vi "configuration UI.vi"() -> ()   [LabVIEW 2014, in "OPC UA Client editor node.lvclass"]
uses:
  OPC UA Client editor node.lvclass
  <vilib>/NI/Configuration Framework/Node/NodeRef.ctl
  <vilib>/NI/Configuration Framework/Node/NISE_CEF_Node.lvclass
  <vilib>/NI/AMC/Message Queue.ctl
  <vilib>/NI/AMC/Message.ctl
  <vilib>/NI/Tools/Keyed Array/KeyedArray.ctl
  <vilib>/NI/Configuration Framework/Node/UserEventRef.ctl
  <vilib>/NI/Configuration Framework/Controls/EventCluster.ctl
  <vilib>/NI/DCAF UI Toolkit/Controls/Configure.ctl
  <vilib>/NI/DCAF UI Toolkit/Controls/Add.ctl
  <vilib>/NI/DCAF UI Toolkit/Controls/Remove.ctl
  <vilib>/NI/Configuration Framework/Node/StopEvent.ctl
  <vilib>/NI/Configuration Framework/Node/RefreshUIEvent.ctl
  <vilib>/NI/Configuration Framework/Node/CacheState.ctl
  <vilib>/NI/Configuration Framework/Node/NodeChangeEvent.ctl
  <vilib>/NI/Tag Bus/tag/Data Type.ctl
  Permissions Enum.ctl
  <vilib>/NI/DCAF/Tag Editor Core/Table API/Available Tag Menu/channel action event.ctl
  <vilib>/NI/DCAF/Tag Editor Core/Table API/Available Tag Menu/dialog output action.ctl
  <vilib>/NI/Tag Bus Module Framework/channel/TBM channel.lvclass
  <vilib>/NI/Tag Bus/tag/tag descriptor.lvclass
  <vilib>/NI/DCAF/Tag Editor Core/Table API/Table Manager/Call Back Ref Type Def.ctl
  <vilib>/NI/DCAF/Tag Editor Core/Configuration Editor/Classes/Engine Parent/Engine Parent Editor Node.lvclass
  <vilib>/NI/DCAF/Tag Editor Core/Configuration Editor/Classes/Module editor node/module editor node.lvclass
  OPC UA DataType Enum.ctl
  <vilib>/NI/DCAF/Tag Editor Core/Table API/Table Manager/references.ctl
  module/configuration/OPC UA Client configuration.lvclass
  module/configuration/OPC UA Client configuration.lvclass/OPC UA Client configuration.ctl
  OPC UA Client editor node.lvclass/OPC UA Client editor node.ctl
  module/configuration/Read Connection Configuration.vi
  module/configuration/Write Connection Configuration.vi
  <vilib>/NI/Configuration Framework/serializable configuration/NISE_CEF_serializable configuration.lvclass
  <vilib>/NI/DCAF/Tag Editor Core/Table API/Listbox/Multi Column Listbox.lvclass
  <vilib>/NI/Configuration Framework/NISE_CEF_TreeControl.lvlib
  <vilib>/NI/Tools/Keyed Array/Tools_KeyedArray.lvlib
  <vilib>/NI/AMC/AMC.lvlib
  <vilib>/NI/DCAF/Tag Editor Core/Table API/Table Manager.lvlib
  <vilib>/NI/DCAF/Tag Editor Core/Table API/Table Manager/Table Manager.lvclass
  <vilib>/NI/DCAF UI Toolkit/Controls/DCAF UI Elements.lvlib
panel:
  in  "OPC Data Type":T1
  in  "user event out":refnum<user-event>
  in  "Permissions":T2
  in  "data type":T3
  in  "node change":T4
  in  "cache state":T5
  in  "refresh UI":T6
  in  "stop event":T7
  in  "Tab Control":enum32{"Nodes", "Client Configuration"}(tab)
  in  "Remove Button":T8
  in  "Add Button":T9
  in  "Table":i32(listbox)
  in  "settings":T10
  in  "ClientCert.Relative?":bool
  in  "ServerCerts.Relative?":bool
  in  "Server Certificate Paths":string[](array[string])
  in  "Client Certificate Path":string
  in  "Server Endpoint URL":string
  in  "Username/Password":cluster{"Username":string, "Password":string}
  in  "Security Policy":T11
  in  "user event":T12
  in  "main queue":T13
  in  "node ref":T14
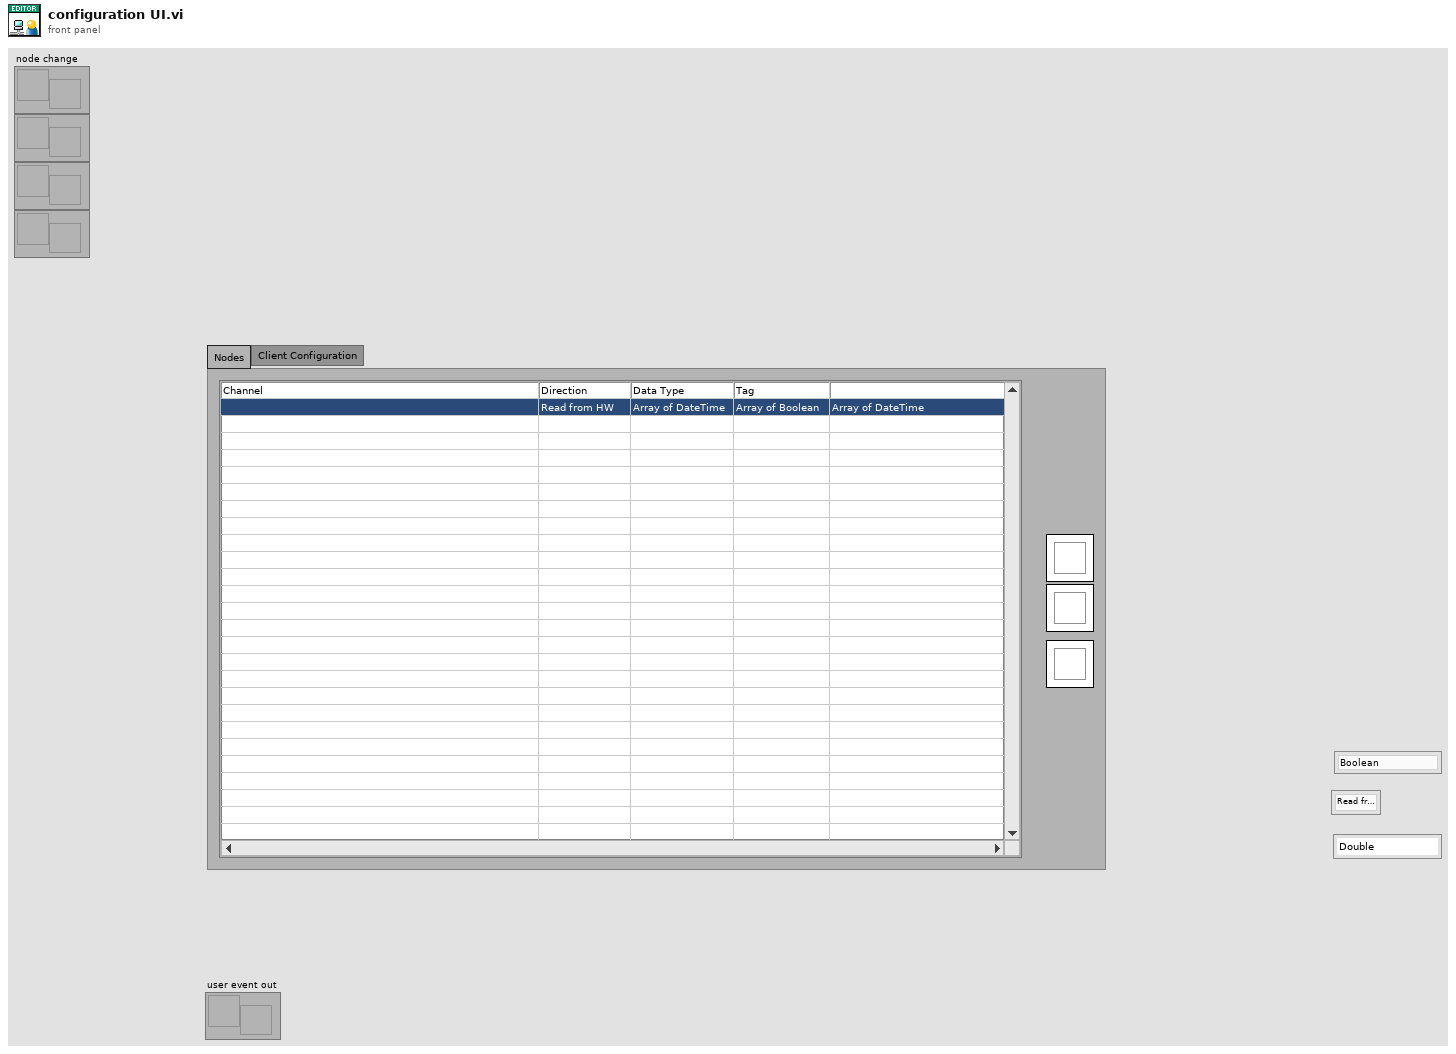
[diagram p1: front panel]
types:
  T1 = typedef "OPC UA Client editor node.lvclass/OPC UA DataType Enum.ctl" = enum16{"Boolean", "SByte", "Byte", "Int16", "UInt16", "Int32", "UInt32", "Int64", "UInt64", "Float", "Double", "String", "DateTime", "ByteString", "Array of Boolean", "Array of SByte", "Array of Byte", "Array of Int16", "Array of UInt16", "Array of Int32", "Array of UInt32", "Array of Int64", "Array of UInt64", "Array of Float", "Array of Double", "Array of String", "Array of DateTime"}
  T2 = typedef "OPC UA Client editor node.lvclass/Permissions Enum.ctl" = enum16{"Read from HW", "Write to HW"}
  T3 = typedef "tag bus.lvlib/tag descriptor.lvclass/Data Type.ctl" = enum16{"Double", "Single", "I64", "I32", "I16", "I8", "U64", "U32", "U16", "U8", "Boolean", "String", "Array of Double", "Array of Single", "Array of I64", "Array of I32", "Array of I16", "Array of I8", "Array of U64", "Array of U32", "Array of U16", "Array of U8", "Array of Boolean", "Array of String"}
  T4 = typedef "NISE_CEF_Node.lvclass/NodeChangeEvent.ctl" = refnum<user-event>
  T5 = typedef "NISE_CEF_Node.lvclass/CacheState.ctl" = refnum<user-event>
  T6 = typedef "NISE_CEF_Node.lvclass/RefreshUIEvent.ctl" = refnum<user-event>
  T7 = typedef "NISE_CEF_Node.lvclass/StopEvent.ctl" = refnum<user-event>
  T8 = typedef "DCAF UI Elements.lvlib/Remove.ctl" = bool
  T9 = typedef "DCAF UI Elements.lvlib/Add.ctl" = bool
  T10 = typedef "DCAF UI Elements.lvlib/Configure.ctl" = bool
  T11 = cluster{"Message Mode":enum16{"None", "Sign", "Sign and Encrypt"}, "Security":enum16{"Basic256", "Basic128Rsa15"}}
  T12 = typedef "NISE_CEF_Node.lvclass/UserEventRef.ctl" = refnum<user-event>
  T13 = typedef "AMC.lvlib/Message Queue.ctl" = refnum<queue>
  T14 = typedef "NISE_CEF_Node.lvclass/NodeRef.ctl" = refnum<data-value>
  T15 = typedef "Table Manager.lvlib/Table Manager.lvclass/references.ctl" = cluster{"stop event":T7, "refresh UI":T6, "cache state":T5, "node change":T4, "user event out":refnum<user-event>, "main queue":T13, "user event":T12}
  T16 = typedef "Table Manager.lvlib/Table Manager.lvclass/object ref.ctl" = cluster{"engine":refnum<data-value>, "Node Ref":refnum<data-value>}
  T17 = typedef "OPC UA Client configuration.lvclass/Client Connection Configuration.ctl" = cluster{"Server Certificates":cluster{"Relative Path?":bool, "Server Paths":string[]}, "Client Certificates":cluster{"Relative Path?":bool, "Client Path":string}, "Client Configuration":cluster{"Server Endpoint URL":string, "Security Policy":cluster{"Message Mode":enum16{"None", "Sign", "Sign and Encrypt"}, "Security":enum16{"Basic256", "Basic128Rsa15"}}, "Username/Password":cluster{"Username":string, "Password":string}}}
  T18 = typedef "Table Manager.lvlib/Column.lvclass/Column Descriptor.ctl" = cluster{"name":string, "caption":string, "Column Type":T19, "Params":string, "AutoSizeMode":i32, "FillWeight":sgl, "MinWidth":u32, "tooltip":string, "Enum Reference":refnum<vi>, "Channel suffix":string, "Read Only":bool, "Call Back VI":T20, "DT Dependency":i32, "name dependency":i32, "data type":T3, "Custom Column":refnum<class "Column.lvclass">}
  T19 = typedef "Table Manager.lvlib/Column.lvclass/Column Type.ctl" = enum16{"String", "Mapping", "Enum", "Custom"}
  T20 = typedef "Table Manager.lvlib/Table Manager.lvclass/Call Back Ref Type Def.ctl" = refnum<vi>
  T21 = typedef "Table Manager.lvlib/Table Manager.lvclass/Table Events.ctl" = cluster{"Menu Selection":refnum<user-event>}
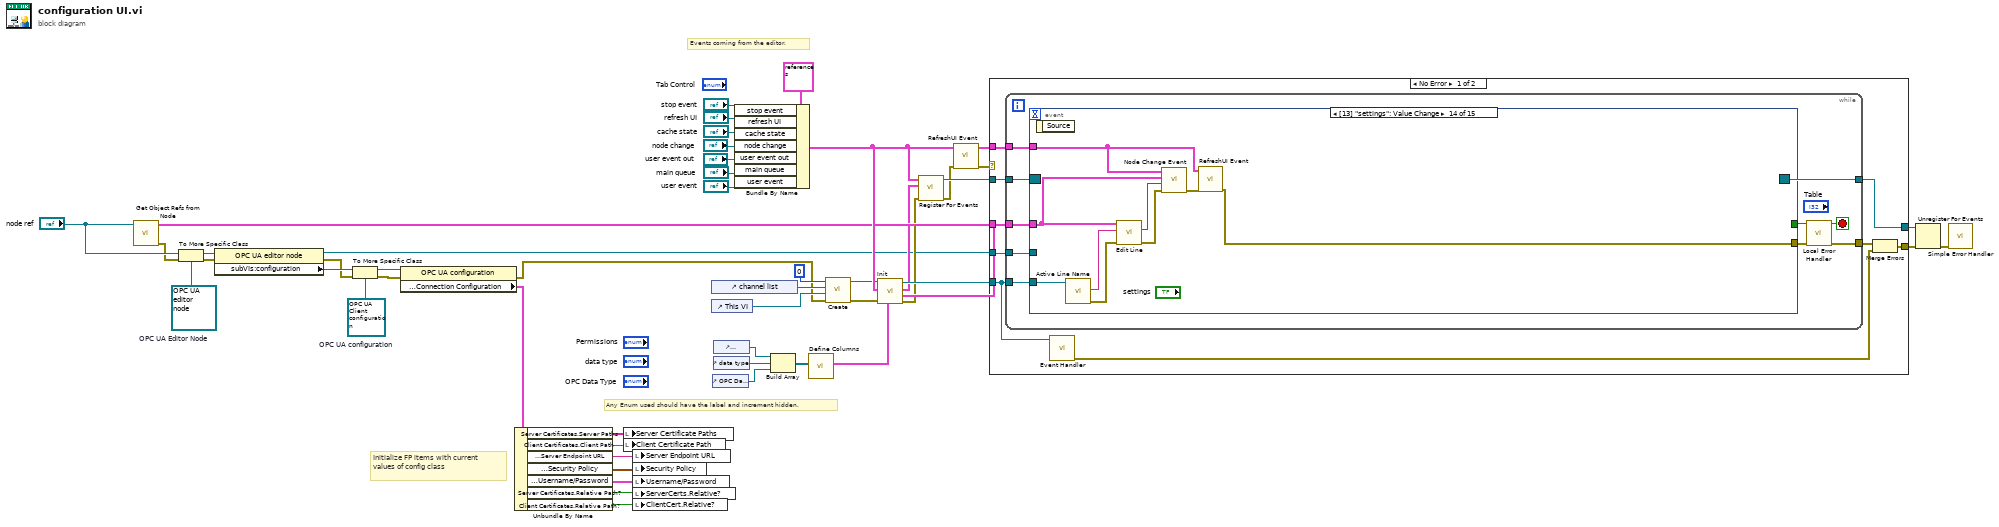
[diagram p0: block diagram]
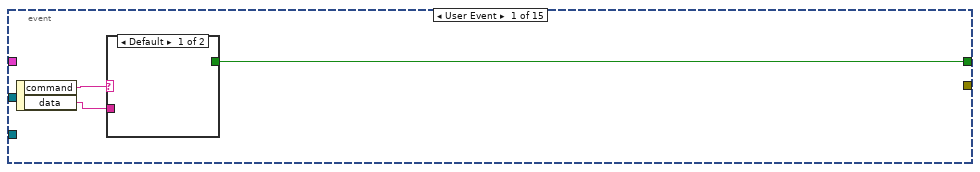
[diagram p2: hidden frame]
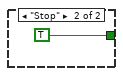
[diagram p3: hidden frame]
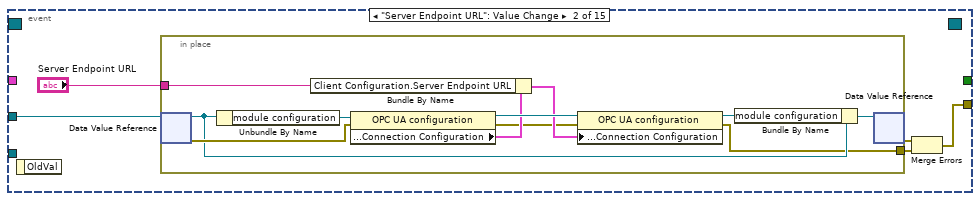
[diagram p4: hidden frame]
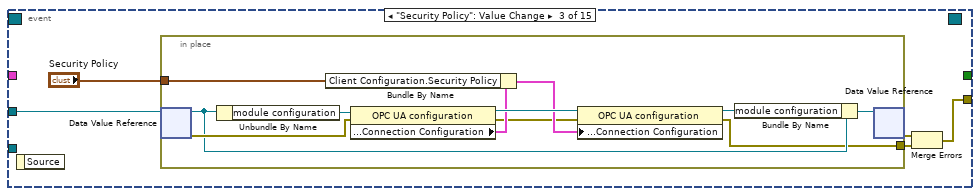
[diagram p5: hidden frame]
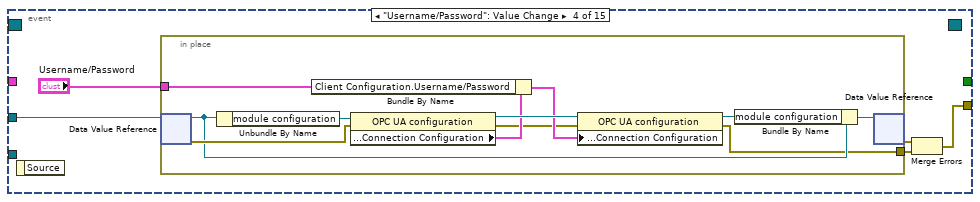
[diagram p6: hidden frame]
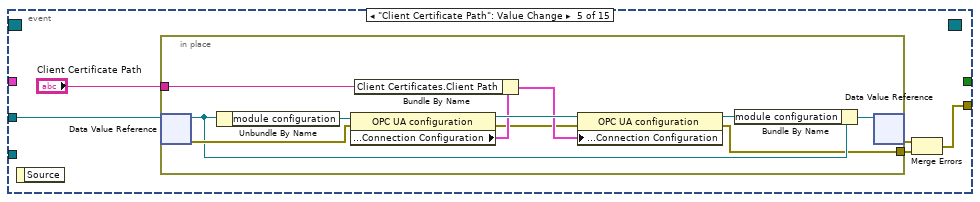
[diagram p7: hidden frame]
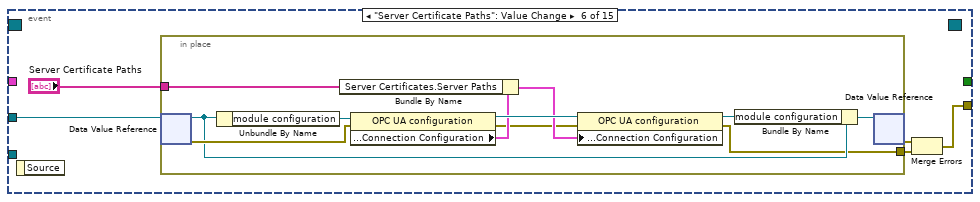
[diagram p8: hidden frame]
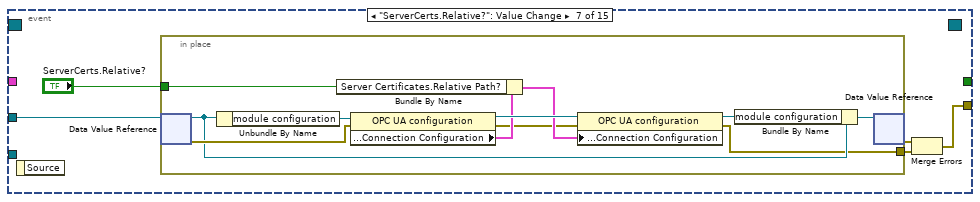
[diagram p9: hidden frame]
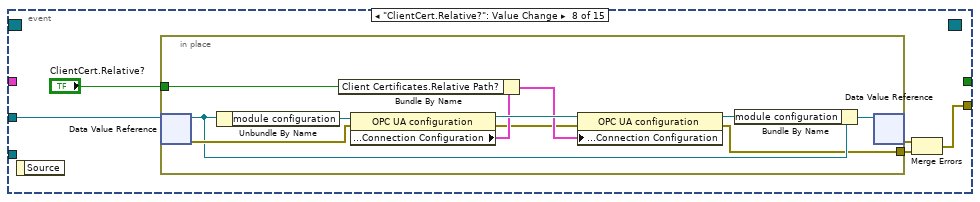
[diagram p10: hidden frame]
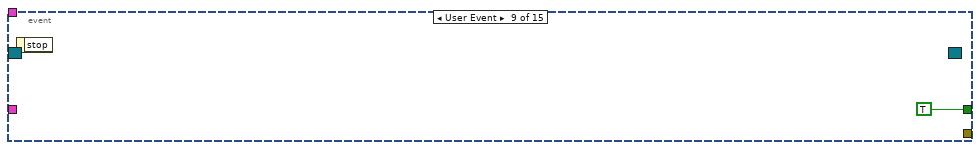
[diagram p11: hidden frame]
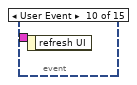
[diagram p12: hidden frame]
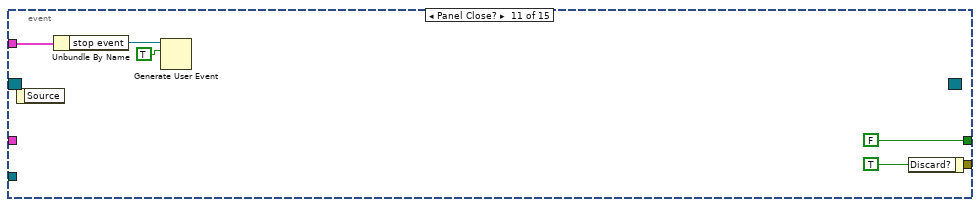
[diagram p13: hidden frame]
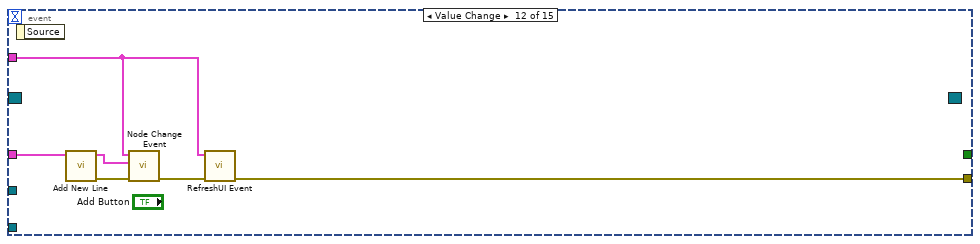
[diagram p14: hidden frame]
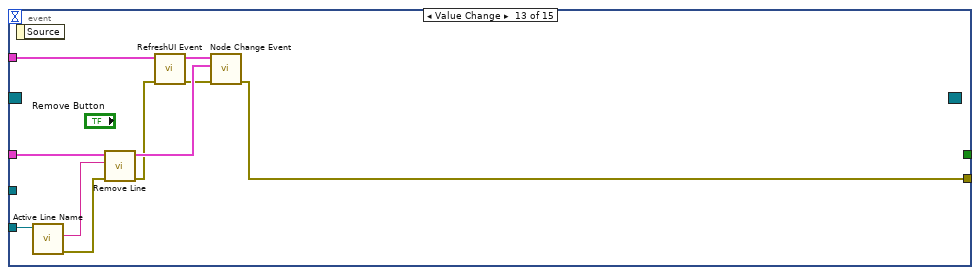
[diagram p15: hidden frame]
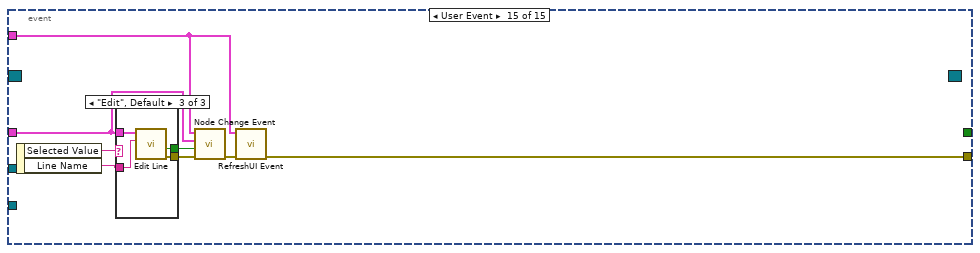
[diagram p16: hidden frame]
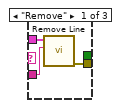
[diagram p17: hidden frame]
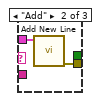
[diagram p18: hidden frame]
diagram:
  w11 = refnum<class "OPC UA Client configuration.lvclass"> refnum  # OPC UA configuration
  w19 = refnum<data-value> refnum  # OPC UA Editor Node
  # "Initialize FP items with current values of config class"
  # "Any Enum used should have the label and increment hidden."
  # "Events coming from the editor."
  n1 = call "Get Object Refs from Node.vi"("Data Value Reference in"="node ref") -> ("error out"=w18:errorcluster, "references"=w32:T16)  [unwired: 9 in]
  n2 = To More Specific Class(target class=w19, reference="node ref", error in=w18) -> (specific class reference=w16:refnum<data-value>, error out=w17:errorcluster)
  n3 = property class="OPC UA editor node"(reference=w16, error in=w17) -> (reference out=w15:refnum<data-value>, error out=w9:errorcluster, "subVIs:configuration"=w14:refnum<class "NISE_CEF_serializable configuration.lvclass">)
  n4 = To More Specific Class(target class=w11, reference=w14, error in=w9) -> (specific class reference=w13:refnum<class "OPC UA Client configuration.lvclass">, error out=w12:errorcluster)
  n5 = property class="OPC UA configuration"(reference=w13, error in=w12) -> (error out=w8:errorcluster, "Customize:Properties:Connection Configuration"=w10:T17)  [unwired: 1 out]
  n6 = Unbundle By Name(w10) -> ("Server Certificates.Server Paths"=w6:string[], "Client Certificates.Client Path"=w5:string, "Client Configuration.Server Endpoint URL"=w2:string, "Client Configuration.Security Policy"=w3:T11, "Client Configuration.Username/Password"=w4:cluster{"Username":string, "Password":string}, "Server Certificates.Relative Path?"=w50:bool, "Client Certificates.Relative Path?"=w1:bool)
  n7 = local write "Server Certificate Paths"(w6) -> ()
  n8 = local write "Client Certificate Path"(w5) -> ()
  n9 = local write "Server Endpoint URL"(w2) -> ()
  n10 = local write "Security Policy"(w3) -> ()
  n11 = local write "Username/Password"(w4) -> ()
  n12 = local write "ServerCerts.Relative?"(w50) -> ()
  n13 = local write "ClientCert.Relative?"(w1) -> ()
  n14 = control-ref of="channel list"() -> (w25:refnum<vi>)
  n15 = control-ref of="This VI"() -> (w23:refnum<vi>)
  n16 = control-ref of="OPC Data Type"() -> (w21:refnum<vi>)
  n17 = control-ref of="Permissions"() -> (w35:refnum<vi>)
  n18 = control-ref of="data type"() -> (w34:refnum<vi>)
  n19 = Bundle By Name(cluster=T15 {"stop event"=refnum, "refresh UI"=refnum, "cache state"=refnum, "node change"=refnum, "user event out"=refnum, "main queue"=refnum, "user event"=refnum} ("References"), "stop event"="stop event", "refresh UI"="refresh UI", "cache state"="cache state", "node change"="node change", "user event out"="user event out", "main queue"="main queue", "user event"="user event") -> (w36:T15)
  n20 = Build Array(w35, w34, w21) -> (w33:refnum<vi>[])
  n21 = call "Define Columns.vi"("Enum Array"=w33) -> ("Column Definition"=w38:T18[])  [unwired: 10 in]
  n22 = call <vilib>:"Create.vi"("error in (no error)"=w8, "Top VI"=w23, "Listbox"=w25, "Index"=0) -> ("error out"=w7:errorcluster, "reference out"=w22:refnum<class "Multi Column Listbox.lvclass">)  [unwired: 6 in]
  n23 = call-dynamic "Init.vi"("Column Descriptors"=w38, "error in (no error)"=w7, "Node object refs"=w32, "Event References"=w36, "Multi Column Listbox in"=w22) -> ("error out"=w27:errorcluster, "Table Events"=w26:T21, "Multi Column Listbox out"=w31:refnum<class "Multi Column Listbox.lvclass">)  [unwired: 4 in]
  n24 = call "Register For Events.vi"("error in"=w27, "Table Events"=w26, "References"=w36) -> ("error out"=w29:errorcluster, "Event Registration Refnum"=w39:refnum<event-registration>)  [unwired: 7 in]
  n25 = call "RefreshUI Event.vi"("error in (no error)"=w29, "References in"=w36) -> ("error out"=w28:errorcluster, "References out"=w37:T15)  [unwired: 8 in]
  n26 = case shown="No Error" w28 {
    selector: w28 -> [_ w233]
    tunnel: w39 -> [w59 w232]
    tunnel: [w58 w232] -> w49
    tunnel: [w52 w233] -> w48
    tunnel: w37 -> [w57 _]
    tunnel: w32 -> [w56 _]
    tunnel: w31 -> [w55 _]
    tunnel: w15 -> [w51 _]
    frame No Error {
      n27 = while {
        tunnel: w59 -> [w69]
        tunnel: [w68] -> w58
        tunnel: [w65] -> w53
        tunnel: w57 -> [w63]
        tunnel: w56 -> [w62]
        tunnel: w55 -> [w61]
        tunnel: w51 -> [w60]
        stop <- w67 stop-if-true
        n28 = event shown="[13] \"settings\": Value Change" {
          selector: w69 -> [_ _ _ _ _ _ _ _ _ _ _ _ _ _ _]
          dyn-events: [_ _ _ _ _ _ _ _ _ _ _ _ _ _ _] -> w68
          timeout: _ -> [_ _ _ _ _ _ _ _ _ _ _ _ _ _ _]
          tunnel: [w72 _ _ _ _ _ _ _ TRUE _ FALSE _ _ _ _] -> w66
          tunnel: [_ w74 w91 w107 w123 w139 w155 w171 _ _ _ w192 w200 w207 w220] -> w64
          tunnel: w63 -> [_ _ _ _ _ _ _ _ _ _ w188 w195 w205 w206 w216]
          tunnel: w62 -> [_ _ _ _ _ _ _ _ _ _ _ w196 w204 w212 w217]
          tunnel: w61 -> [_ _ _ _ _ _ _ _ _ _ _ _ w199 w213 _]
          tunnel: w60 -> [_ w78 w94 w110 w126 w142 w158 w174 _ _ _ _ _ _ _]
          event User Event {
            n29 = event-data() -> ("command"=w71:string, "data"=w70:string)  [unwired: 1 in]
            n30 = case shown="Default" w71 {
              tunnel: [_ TRUE] -> w72
              tunnel: w70 -> [_ _]
              frame Default {
              }
              frame "Stop" {
              }
            }
          }
          event "Server Endpoint URL": Value Change {
            n31 = event-data() -> ()  [unwired: 1 in, 1 out]
            n32 = in-place {
              in-place-border: "Server Endpoint URL" -> [w85]
              in-place-border: [w79] -> w75
              n33 = in-place-dvr #1(w78) -> (w81:refnum<class "OPC UA Client editor node.lvclass">, w84:errorcluster)
              n34 = Unbundle By Name(w81) -> ("module configuration"=w89:refnum<class "OPC UA Client configuration.lvclass">)
              n35 = property class="OPC UA configuration"(reference=w89, error in=w84) -> (reference out=w88:refnum<class "OPC UA Client configuration.lvclass">, error out=w83:errorcluster, "Customize:Properties:Connection Configuration"=w87:T17)
              n36 = Bundle By Name(cluster=w87, "Client Configuration.Server Endpoint URL"=w85) -> (w86:T17)
              n37 = property class="OPC UA configuration"(reference=w88, error in=w83, "Customize:Properties:Connection Configuration"=w86) -> (reference out=w82:refnum<class "OPC UA Client configuration.lvclass">, error out=w79:errorcluster)
              n38 = Bundle By Name(cluster=w81, "module configuration"=w82) -> (w80:refnum<class "OPC UA Client editor node.lvclass">)
              n39 = in-place-dvr #1(w80) -> (w76:errorcluster)  [unwired: 1 out]
            }
            n40 = Merge Errors(w76, w75) -> (w74:errorcluster)
          }
          event "Security Policy": Value Change {
            n41 = event-data() -> ()  [unwired: 1 in, 1 out]
            n42 = in-place {
              in-place-border: "Security Policy" -> [w101]
              in-place-border: [w95] -> w92
              n43 = in-place-dvr #2(w94) -> (w97:refnum<class "OPC UA Client editor node.lvclass">, w100:errorcluster)
              n44 = Unbundle By Name(w97) -> ("module configuration"=w105:refnum<class "OPC UA Client configuration.lvclass">)
              n45 = property class="OPC UA configuration"(reference=w105, error in=w100) -> (reference out=w104:refnum<class "OPC UA Client configuration.lvclass">, error out=w99:errorcluster, "Customize:Properties:Connection Configuration"=w103:T17)
              n46 = Bundle By Name(cluster=w103, "Client Configuration.Security Policy"=w101) -> (w102:T17)
              n47 = property class="OPC UA configuration"(reference=w104, error in=w99, "Customize:Properties:Connection Configuration"=w102) -> (reference out=w98:refnum<class "OPC UA Client configuration.lvclass">, error out=w95:errorcluster)
              n48 = Bundle By Name(cluster=w97, "module configuration"=w98) -> (w96:refnum<class "OPC UA Client editor node.lvclass">)
              n49 = in-place-dvr #2(w96) -> (w93:errorcluster)  [unwired: 1 out]
            }
            n50 = Merge Errors(w93, w92) -> (w91:errorcluster)
          }
          event "Username/Password": Value Change {
            n51 = event-data() -> ()  [unwired: 1 in, 1 out]
            n52 = in-place {
              in-place-border: "Username/Password" -> [w117]
              in-place-border: [w111] -> w108
              n53 = in-place-dvr #3(w110) -> (w113:refnum<class "OPC UA Client editor node.lvclass">, w116:errorcluster)
              n54 = Unbundle By Name(w113) -> ("module configuration"=w121:refnum<class "OPC UA Client configuration.lvclass">)
              n55 = property class="OPC UA configuration"(reference=w121, error in=w116) -> (reference out=w120:refnum<class "OPC UA Client configuration.lvclass">, error out=w115:errorcluster, "Customize:Properties:Connection Configuration"=w119:T17)
              n56 = Bundle By Name(cluster=w119, "Client Configuration.Username/Password"=w117) -> (w118:T17)
              n57 = property class="OPC UA configuration"(reference=w120, error in=w115, "Customize:Properties:Connection Configuration"=w118) -> (reference out=w114:refnum<class "OPC UA Client configuration.lvclass">, error out=w111:errorcluster)
              n58 = Bundle By Name(cluster=w113, "module configuration"=w114) -> (w112:refnum<class "OPC UA Client editor node.lvclass">)
              n59 = in-place-dvr #3(w112) -> (w109:errorcluster)  [unwired: 1 out]
            }
            n60 = Merge Errors(w109, w108) -> (w107:errorcluster)
          }
          event "Client Certificate Path": Value Change {
            n61 = event-data() -> ()  [unwired: 1 in, 1 out]
            n62 = in-place {
              in-place-border: "Client Certificate Path" -> [w133]
              in-place-border: [w127] -> w124
              n63 = in-place-dvr #4(w126) -> (w129:refnum<class "OPC UA Client editor node.lvclass">, w132:errorcluster)
              n64 = Unbundle By Name(w129) -> ("module configuration"=w137:refnum<class "OPC UA Client configuration.lvclass">)
              n65 = property class="OPC UA configuration"(reference=w137, error in=w132) -> (reference out=w136:refnum<class "OPC UA Client configuration.lvclass">, error out=w131:errorcluster, "Customize:Properties:Connection Configuration"=w135:T17)
              n66 = Bundle By Name(cluster=w135, "Client Certificates.Client Path"=w133) -> (w134:T17)
              n67 = property class="OPC UA configuration"(reference=w136, error in=w131, "Customize:Properties:Connection Configuration"=w134) -> (reference out=w130:refnum<class "OPC UA Client configuration.lvclass">, error out=w127:errorcluster)
              n68 = Bundle By Name(cluster=w129, "module configuration"=w130) -> (w128:refnum<class "OPC UA Client editor node.lvclass">)
              n69 = in-place-dvr #4(w128) -> (w125:errorcluster)  [unwired: 1 out]
            }
            n70 = Merge Errors(w125, w124) -> (w123:errorcluster)
          }
          event "Server Certificate Paths": Value Change {
            n71 = event-data() -> ()  [unwired: 1 in, 1 out]
            n72 = in-place {
              in-place-border: "Server Certificate Paths" -> [w149]
              in-place-border: [w143] -> w140
              n73 = in-place-dvr #5(w142) -> (w145:refnum<class "OPC UA Client editor node.lvclass">, w148:errorcluster)
              n74 = Unbundle By Name(w145) -> ("module configuration"=w153:refnum<class "OPC UA Client configuration.lvclass">)
              n75 = property class="OPC UA configuration"(reference=w153, error in=w148) -> (reference out=w152:refnum<class "OPC UA Client configuration.lvclass">, error out=w147:errorcluster, "Customize:Properties:Connection Configuration"=w151:T17)
              n76 = Bundle By Name(cluster=w151, "Server Certificates.Server Paths"=w149) -> (w150:T17)
              n77 = property class="OPC UA configuration"(reference=w152, error in=w147, "Customize:Properties:Connection Configuration"=w150) -> (reference out=w146:refnum<class "OPC UA Client configuration.lvclass">, error out=w143:errorcluster)
              n78 = Bundle By Name(cluster=w145, "module configuration"=w146) -> (w144:refnum<class "OPC UA Client editor node.lvclass">)
              n79 = in-place-dvr #5(w144) -> (w141:errorcluster)  [unwired: 1 out]
            }
            n80 = Merge Errors(w141, w140) -> (w139:errorcluster)
          }
          event "ServerCerts.Relative?": Value Change {
            n81 = event-data() -> ()  [unwired: 1 in, 1 out]
            n82 = in-place {
              in-place-border: "ServerCerts.Relative?" -> [w165]
              in-place-border: [w159] -> w156
              n83 = in-place-dvr #6(w158) -> (w161:refnum<class "OPC UA Client editor node.lvclass">, w164:errorcluster)
              n84 = Unbundle By Name(w161) -> ("module configuration"=w169:refnum<class "OPC UA Client configuration.lvclass">)
              n85 = property class="OPC UA configuration"(reference=w169, error in=w164) -> (reference out=w168:refnum<class "OPC UA Client configuration.lvclass">, error out=w163:errorcluster, "Customize:Properties:Connection Configuration"=w167:T17)
              n86 = Bundle By Name(cluster=w167, "Server Certificates.Relative Path?"=w165) -> (w166:T17)
              n87 = property class="OPC UA configuration"(reference=w168, error in=w163, "Customize:Properties:Connection Configuration"=w166) -> (reference out=w162:refnum<class "OPC UA Client configuration.lvclass">, error out=w159:errorcluster)
              n88 = Bundle By Name(cluster=w161, "module configuration"=w162) -> (w160:refnum<class "OPC UA Client editor node.lvclass">)
              n89 = in-place-dvr #6(w160) -> (w157:errorcluster)  [unwired: 1 out]
            }
            n90 = Merge Errors(w157, w156) -> (w155:errorcluster)
          }
          event "ClientCert.Relative?": Value Change {
            n91 = event-data() -> ()  [unwired: 1 in, 1 out]
            n92 = in-place {
              in-place-border: "ClientCert.Relative?" -> [w181]
              in-place-border: [w175] -> w172
              n93 = in-place-dvr #7(w174) -> (w177:refnum<class "OPC UA Client editor node.lvclass">, w180:errorcluster)
              n94 = Unbundle By Name(w177) -> ("module configuration"=w185:refnum<class "OPC UA Client configuration.lvclass">)
              n95 = property class="OPC UA configuration"(reference=w185, error in=w180) -> (reference out=w184:refnum<class "OPC UA Client configuration.lvclass">, error out=w179:errorcluster, "Customize:Properties:Connection Configuration"=w183:T17)
              n96 = Bundle By Name(cluster=w183, "Client Certificates.Relative Path?"=w181) -> (w182:T17)
              n97 = property class="OPC UA configuration"(reference=w184, error in=w179, "Customize:Properties:Connection Configuration"=w182) -> (reference out=w178:refnum<class "OPC UA Client configuration.lvclass">, error out=w175:errorcluster)
              n98 = Bundle By Name(cluster=w177, "module configuration"=w178) -> (w176:refnum<class "OPC UA Client editor node.lvclass">)
              n99 = in-place-dvr #7(w176) -> (w173:errorcluster)  [unwired: 1 out]
            }
            n100 = Merge Errors(w173, w172) -> (w171:errorcluster)
          }
          event User Event {
            n101 = event-data() -> ()  [unwired: 1 in, 1 out]
          }
          event User Event {
            n102 = event-data() -> ()  [unwired: 1 in, 1 out]
          }
          event Panel Close? {
            n103 = event-data() -> ()  [unwired: 1 in, 1 out]
            n104 = Unbundle By Name(w188) -> ("stop event"=w187:T7)
            n105 = Generate User Event(user event=w187, event data cluster=TRUE ("event data")) -> ()  [unwired: 2 in, 2 out]
            n106 = event-data("Discard?"=TRUE) -> ()  [unwired: 1 in, 1 out]
          }
          event Value Change {
            n107 = event-data() -> ()  [unwired: 1 in, 1 out]
            n108 = call "Add New Line.vi"("objects"=w196) -> ("error out"=w194:errorcluster)  [unwired: 9 in, 1 out]
            n109 = call "Node Change Event.vi"("error in (no error)"=w194, "objects"=w196, "References in"=w195) -> ("error out"=w193:errorcluster)  [unwired: 8 in]
            n110 = call "RefreshUI Event.vi"("error in (no error)"=w193, "References in"=w195) -> ("error out"=w192:errorcluster)  [unwired: 8 in, 1 out]
          }
          event Value Change {
            n111 = event-data() -> ()  [unwired: 1 in, 1 out]
            n112 = call-dynamic "Active Line Name.vi"("Multi Column Listbox in"=w199) -> ("error out"=w197:errorcluster, "Active Line Name"=w198:string)  [unwired: 8 in, 1 out]
            n113 = call "Remove Line.vi"("error in"=w197, "Active Line Name"=w198, "Objects"=w204) -> ("error out"=w201:errorcluster)  [unwired: 8 in]
            n114 = call "RefreshUI Event.vi"("error in (no error)"=w201, "References in"=w205) -> ("error out"=w203:errorcluster, "References out"=w202:T15)  [unwired: 8 in]
            n115 = call "Node Change Event.vi"("error in (no error)"=w203, "objects"=w204, "References in"=w202) -> ("error out"=w200:errorcluster)  [unwired: 8 in]
          }
          event Value Change {
            n116 = event-data() -> ()  [unwired: 1 in, 1 out]
            n117 = call-dynamic "Active Line Name.vi"("Multi Column Listbox in"=w213) -> ("error out"=w210:errorcluster, "Active Line Name"=w211:string)  [unwired: 8 in, 1 out]
            n118 = call "Edit Line.vi"("error in"=w210, "Line Name"=w211, "References"=w212) -> ("error out"=w214:errorcluster, "change?"=w209:bool)  [unwired: 7 in]
            n119 = call "Node Change Event.vi"("error in (no error)"=w214, "Send"=w209, "objects"=w212, "References in"=w206) -> ("error out"=w208:errorcluster)  [unwired: 7 in]
            n120 = call "RefreshUI Event.vi"("error in (no error)"=w208, "References in"=w206) -> ("error out"=w207:errorcluster)  [unwired: 8 in, 1 out]
          }
          event User Event {
            n121 = event-data() -> ("Selected Value"=w222:string, "Line Name"=w219:string)  [unwired: 1 in]
            n122 = case shown="\"Edit\", Default" w222 {
              tunnel: w219 -> [w225 _ w231]
              tunnel: w217 -> [w224 w227 w230]
              tunnel: [w223 w226 w229] -> w218
              tunnel: [_ _ w228] -> w215
              frame "Remove" {
                n123 = call "Remove Line.vi"("Active Line Name"=w225, "Objects"=w224) -> ("error out"=w223:errorcluster)  [unwired: 9 in]
              }
              frame "Add" {
                n124 = call "Add New Line.vi"("objects"=w227) -> ("error out"=w226:errorcluster)  [unwired: 9 in, 1 out]
              }
              frame "Edit", Default {
                n125 = call "Edit Line.vi"("Line Name"=w231, "References"=w230) -> ("error out"=w229:errorcluster, "change?"=w228:bool)  [unwired: 8 in]
              }
            }
            n126 = call "Node Change Event.vi"("error in (no error)"=w218, "Send"=w215, "objects"=w217, "References in"=w216) -> ("error out"=w221:errorcluster)  [unwired: 7 in]
            n127 = call "RefreshUI Event.vi"("error in (no error)"=w221, "References in"=w216) -> ("error out"=w220:errorcluster)  [unwired: 8 in, 1 out]
          }
        }
        n128 = call "Local Error Handler.vi"("error in"=w64, "Stop in"=w66) -> ("error out"=w65:errorcluster, "Stop out"=w67:bool)  [unwired: 8 in]
      }
      n129 = call-dynamic "Event Handler.vi"("Listbox in"=w55) -> ("error out"=w54:errorcluster)  [unwired: 9 in, 1 out]
      n130 = Merge Errors(w53, w54) -> (w52:errorcluster)
    }
    frame Error {
    }
  }
  n131 = Unregister For Events(event registration refnum=w49, error in=w48) -> (error out=w47:errorcluster)
  n132 = call <vilib>:"Simple Error Handler.vi"("error in (no error)"=w47) -> ()  [unwired: 4 in, 5 out]
